vi "Format Generic Data to XML Value.vi"(5 "spaces per level":i32, 6 "level":i32, 7 "Type Formatting":T1, 8 "error in (no error)":errorcluster, 9 "attribute? (F: entity)":bool, 11 "LabVIEW Data":variant) -> (0 "error out":errorcluster, 1 "name":string, 2 "value":string, 3 "Data Elements":string)   [LabVIEW 2013]
uses:
  Options API/Private/EasyXML Options - Type Formatting Cluster.ctl
  Type Defs/Formatting Data Type -- Enum.ctl
panel:
  # "OpenG Format Generic Data to XML Value.vi  - formats the data of scalar data\n\nCopyright (C) 2004, 2003 Jim Kring jim@jimkring.com\nCopyright (C) 2004 Ian Dees undees@users.sourceforge.net\n\nThis library is free software; you can redistribute it and/or\nmodify it under the terms of the GNU Lesser General Public\nLicense as published by the Free Software Foundation; either\nversion 2.1 of the License, or (at your option) any later version.\nThis library is distributed in the hope that it will be useful,\nbut WITHOUT ANY WARRANTY; without even the implied warranty of\nMERCHANTABILITY or FITNESS FOR A PARTICULAR PURPOSE. See the GNU\nLesser General Public License for more details.\nYou should have received a copy of the GNU Lesser General Public\nLicense along with this library; if not, write to the Free Software\nFoundation, Inc., 59 Temple Place, Suite 330, Boston, MA 02111-1307 USA"
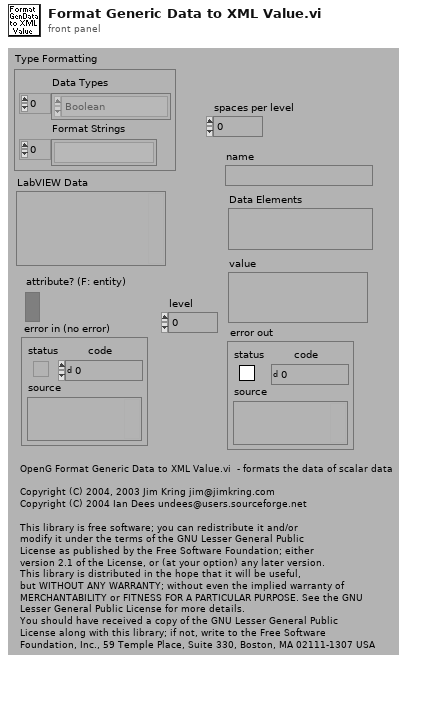
[diagram p1: front panel]
types:
  T1 = typedef "EasyXML Options - Type Formatting Cluster.ctl" = cluster{"Data Types":T2[], "Format Strings":string[]}
  T2 = typedef "Formatting Data Type -- Enum.ctl" = enum16{"<unknown>", "Cluster", "Array", "String", "Path", "Boolean", "Time Stamp", "Enum", "Numeric - EXT", "Numeric - DBL", "Numeric - SGL", "Numeric - I64", "Numeric - I32", "Numeric - I16", "Numeric - I8", "Numeric - U64", "Numeric - U32", "Numeric - U16", "Numeric - U8", "Numeric - CXT", "Numeric - CDB", "Numeric - CSG", "VISA Resource"}
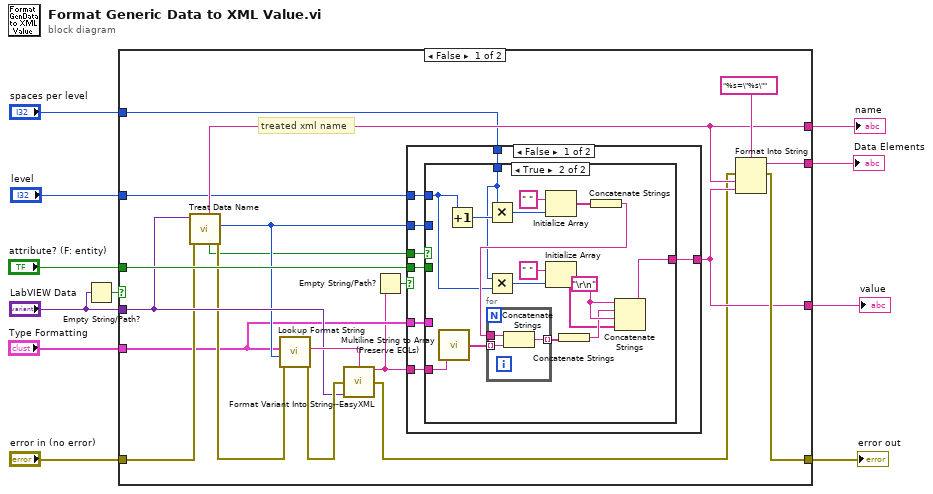
[diagram p0: block diagram]
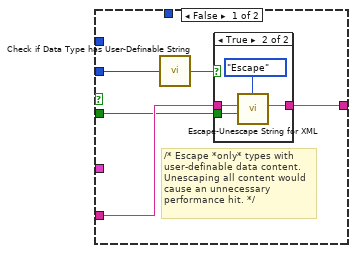
[diagram p2: hidden frame]
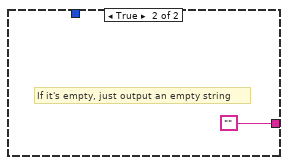
[diagram p4: hidden frame]
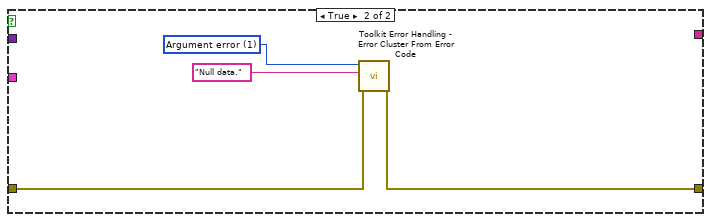
[diagram p5: hidden frame]
diagram:
  n1 = Empty String/Path?(string/path="LabVIEW Data") -> (empty?=w7:bool)
  n2 = case shown="False" w7 {
    tunnel: "LabVIEW Data" -> [w23 _]
    tunnel: "error in (no error)" -> [w19 w70]
    tunnel: [w27 w69] -> w10
    tunnel: [w28 _] -> w9
    tunnel: "Type Formatting" -> [w16 _]
    tunnel: [w26 _] -> w5
    tunnel: [w22 _] -> w4
    tunnel: "attribute? (F: entity)" -> [w24 _]
    tunnel: "level" -> [w14 _]
    tunnel: "spaces per level" -> [w15 _]
    frame False {
      # "treated xml name"
      n3 = call "Treat Data Name.vi"("error in (no error)"=w19, "Data"=w23) -> ("error out"=w18:errorcluster, "EasyXML Type"=w20:T2, "contains raw xml?"=w17:bool, "treated xml name"=w22:string)  [unwired: 3 in, 3 out]
      n4 = call "Lookup Format String.vi"("error in"=w18, "element"=w20, "Type Formatting"=w16) -> ("error out"=w25:errorcluster, "Format String"=w30:string)  [unwired: 5 in, 2 out]
      n5 = call "Format Variant Into String--EasyXML.vi"("format string"=w30, "error in (no error)"=w25, "Variant"=w23) -> ("Output String"=w12:string, "error out"=w21:errorcluster)  [unwired: 11 in]
      n6 = Empty String/Path?(string/path=w12) -> (empty?=w13:bool)
      n7 = case shown="False" w13 {
        tunnel: w12 -> [w38 _]
        tunnel: [w37 "" ("String out")] -> w26
        tunnel: w24 -> [w36 _]
        tunnel: w20 -> [w35 _]
        tunnel: w17 -> [w34 _]
        tunnel: w16 -> [w33 _]
        tunnel: w15 -> [w32 _]
        tunnel: w14 -> [w31 _]
        frame False {
          n8 = case shown="True" w34 {
            tunnel: w38 -> [w42 w56]
            tunnel: [w41 w63] -> w37
            tunnel: w36 -> [w40 _]
            tunnel: w35 -> [w39 _]
            tunnel: w33 -> [_ _]
            tunnel: w32 -> [_ w51]
            tunnel: w31 -> [_ w50]
            frame False {
              # "/* Escape *only* types with user-definable data content. Unescaping all content would cause an unnecessary performance hit. */"
              n9 = call "Check if Data Type has User-Definable String.vi"("EasyXML Type"=w39) -> ("Has User-Definable String Data?"=w43:bool)
              n10 = case shown="True" w43 {
                tunnel: w42 -> [w44 w47]
                tunnel: [w44 w46] -> w41
                tunnel: w40 -> [_ w45]
                frame False {
                }
                frame True {
                  n11 = call "Escape-Unescape String for XML.vi"("attribute? (F: entity)"=w45, "String"=w47, "Action (Escape)"=enum16{"Escape", "Unescape"}."Escape") -> ("String out"=w46:string)  [unwired: 8 in]
                }
              }
            }
            frame True {
              w64 = "\r\n"
              n12 = call "Multiline String to Array (Preserve EOLs).vi"("Input String"=w56) -> ("Array"=w58:string[])
              n13 = Increment(x=w50) -> (x+1=w59:i32)
              n14 = Multiply(x=w51, y=w59) -> (x*y=w61:i32)
              n15 = Multiply(x=w51, y=w50) -> (x*y=w52:i32)
              n16 = Initialize Array(" " ("delimiter (Tab)"), w61) -> (w62:string[])
              n17 = Initialize Array(" " ("delimiter (Tab)"), w52) -> (w49:string[])
              n18 = Concatenate Strings(w62) -> (w54:string)
              n19 = for {
                tunnel: w54 -> [w67]
                tunnel: [w66] -> w57 mode=indexing
                tunnel: w58 -> [w65] mode=indexing
                n20 = Concatenate Strings(w67, w65) -> (w66:string)
              }
              n21 = Concatenate Strings(w57) -> (w55:string)
              n22 = Concatenate Strings(w64, w55, w64, w49) -> (w63:string)
            }
          }
        }
        frame True {
          # "If it's empty, just output an empty string"
        }
      }
      n23 = Format Into String(format string="%s=\"%s\"", error in=w21, w22, w26) -> (resulting string=w28:string, error out=w27:errorcluster)  [unwired: 1 in]
    }
    frame True {
      w72 = 1 items=["No error", "Argument error", "Memory is full", "Out of zone", "End of file", "File already open", "Generic file I/O error", "File not found", "File permission error", "Disk is full", "Duplicate path", "Too many files open", "System feature not enabled", "Resource file not found", "Cannot add resource", "Resource not found", "Image not found", "Image memory error", "Pen does not exist", "Config type invalid", "Config token not found", "Config parse error", "Config memory error", "Bad external code format", "Bad external code offset", "External code not present", "Null window", "Destroy window error", "Null menu", "Print aborted", "Bad print record", "Print driver error", "Windows error during printing", "Memory error during printing", "Print dialog error", "Generic print error", "Invalid device refnum", "Device not found", "Device parameter error", "Device unit error", "Cannot open device", "Device call aborted", "Generic error", "Cancelled by user", "Object ID too low", "Object ID too high", "Object not in heap", "Unknown heap", "Unknown object (invalid DefProc)", "Unknown object (DefProc not in table)", "Message out of range", "Invalid (null) method", "Unknown message", "Manager call not supported", "Bad address", "Network operation in progress", "Network operation timed out", "Connection is busy", "Network attribute not supported", "Network error", "Address in use", "System out of memory", "Connection aborted", "Connection refused", "Not connected", "Already connected", "Connection closed", "Initialization error (interapplication manager)", "Bad occurrence", "Wait on unbound occurrence handler", "Occurrence queue overflow", "Datalog type conflict", "Unused", "Unrecognized type (interapplication manager)", "Memory corrupt", "Failed to make temporary DLL", "Old CIN version", "Drag socket not found", "Failed to load drop-object", "Failed to register OLE object", "Failed to release OLE object", "Format specifier type mismatch", "Unknown format specifier", "Too few format specifiers", "Too many format specifiers", "Scan failed", "Newer CIN version", "Error converting to variant", "Runtime menu error", "Password tampered", "Variant attribute not found", "Incompatible variant data type", "Event data is not available", "Event Store is not present", "Occurrence is not found", "Event Queue is not created", "Event info is not available", "Refnum passed is NULL", "Error retrieving Class GUID", "Error retrieving CoClass GUID", "Error retrieving TypeLib GUID.", "Bad built application magic bytes.", "Specific driver is different from the specific driver associated with the Logical Name.", "There is no session opened to the class driver.", "Max Error", "MAX - Error with config objects", "MAX - Error loading configuration", "MAX - Group not supported"]
      n24 = call "Toolkit Error Handling - Error Cluster From Error Code.vi"("error in"=w70, "error message (\"\")"="Null data." ("error message (\"\")"), "error code (0)"=w72) -> ("error out"=w69:errorcluster)  [unwired: 6 in]
    }
  }
  "error out" <- w10
  "Data Elements" <- w9
  "value" <- w5
  "name" <- w4
